vi "Do[Core].vi"(0 "ControlAction in":refnum<class "GetControlValue.lvclass">, 5 "Ctl Refnum in":refnum<vi>, 11 "error in (no error)":errorcluster) -> (4 "ControlAction out":refnum<class "GetControlValue.lvclass">, 6 "Ctl Refnum out":refnum<vi>, 15 "error out":errorcluster)   [LabVIEW 2016, in "GetControlValue.lvclass"]
uses:
  GetControlValue.lvclass
  GetControlValue.lvclass/GetControlValue.ctl
  VIActionBase/ControlActionBase.lvclass
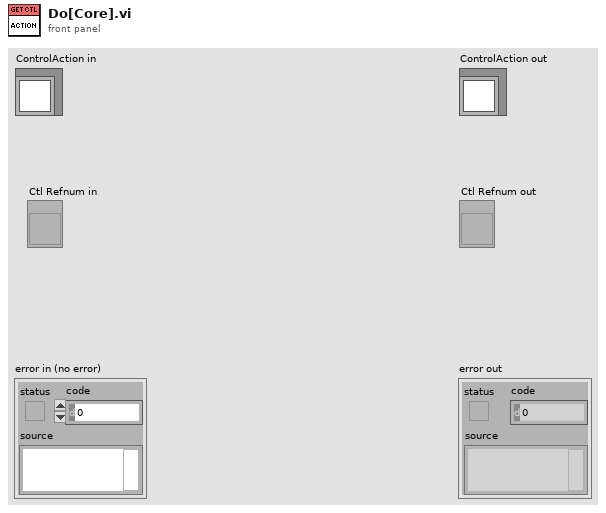
[diagram p1: front panel]
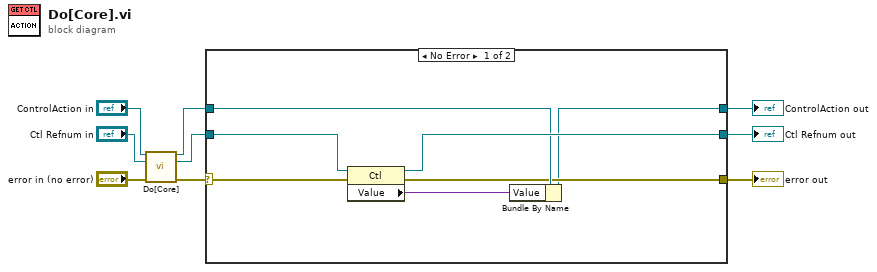
[diagram p0: block diagram]
diagram:
  n1 = call-parent "Do[Core].vi"("ControlAction in"="ControlAction in", "Ctl Refnum in"="Ctl Refnum in", "error in (no error)"="error in (no error)") -> ("ControlAction out"=w1:refnum<class "GetControlValue.lvclass">, "Ctl Refnum out"=w2:refnum<vi>, "error out"=w3:errorcluster)  [unwired: 10 in]
  n2 = case shown="No Error" w3 {
    selector: w3 -> [w14 w19]
    tunnel: [w13 w19] -> w6
    tunnel: [w16 w18] -> w5
    tunnel: [w11 w17] -> w4
    tunnel: w2 -> [w12 w18]
    tunnel: w1 -> [w15 w17]
    frame No Error {
      n3 = property class="Ctl"(reference=w12, error in=w14) -> (reference out=w16:refnum<vi>, error out=w13:errorcluster, "Value"=w10:variant)
      n4 = Bundle By Name(cluster=w15, "Value"=w10) -> (w11:refnum<class "GetControlValue.lvclass">)
    }
    frame Error {
    }
  }
  "error out" <- w6
  "ControlAction out" <- w4
  "Ctl Refnum out" <- w5
